vi "Save_to_Project.vi"(8 "error in (no error)":errorcluster, 9 "index":string, 10 "buildObject":T1, 11 "absFolder in":refnum<class "absFolder.lvclass">) -> (0 "error out":errorcluster, 1 "index out":string, 2 "buildObject out":T1, 3 "absFolder out":refnum<class "absFolder.lvclass">, 5 "saved?":bool)   [LabVIEW 2020, in "absFolder.lvclass"]
uses:
  <vilib>/AppBuilder/IB_Classes/Destination/absFolder/absFolder.lvclass
  <vilib>/AppBuilder/IB_Classes/Destination/absFolder/absFolder.lvclass/absFolder.ctl
  <vilib>/AppBuilder/IB_Classes/Destination/IB_Destination.lvclass
  <vilib>/AppBuilder/IB_RW_Project/IB_RW_Project_PropBag_Action.ctl
  <resource>/Framework/Providers/API/ItemRef.ctl
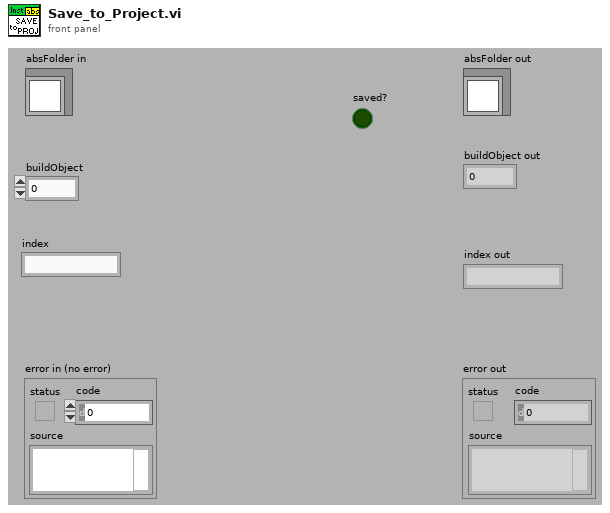
[diagram p1: front panel]
types:
  T1 = typedef "ItemRef.ctl" = u64
  T2 = typedef "IB_RW_Project_PropBag_Action.ctl" = enum16{"read", "write", "clear", "readPrevious", "writePrevious", "clearPrevious"}
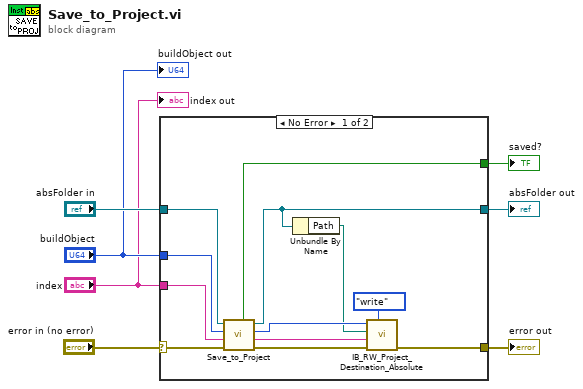
[diagram p0: block diagram]
diagram:
  n1 = case shown="No Error" "error in (no error)" {
    selector: "error in (no error)" -> [w8 w21]
    tunnel: [w19 _] -> w7
    tunnel: "index" -> [w18 _]
    tunnel: "buildObject" -> [w17 _]
    tunnel: "absFolder in" -> [w16 w20]
    tunnel: [w15 w20] -> w5
    tunnel: [w12 w21] -> w4
    frame No Error {
      n2 = call-parent "Save_to_Project.vi"("error in (no error)"=w8, "index"=w18, "buildObject"=w17, "IB_Destination in"=w16) -> ("error out"=w13:errorcluster, "index out"=w10:string, "buildObject out"=w11:T1, "IB_Destination out"=w15:refnum<class "absFolder.lvclass">, "saved?"=w19:bool)  [unwired: 3 in]
      n3 = Unbundle By Name(w15) -> ("Path"=w9:path)
      n4 = call <vilib>:"IB_RW_Project_Destination_Absolute.vi"("action"=IB_RW_Project_PropBag_Action."write", "ErrIn"=w13, "index"=w10, "Path"=w9, "buildObject"=w11) -> ("ErrOut"=w12:errorcluster)  [unwired: 3 in, 3 out]
    }
    frame Error {
    }
  }
  "error out" <- w4
  "absFolder out" <- w5
  "saved?" <- w7
  "buildObject out" <- "buildObject"
  "index out" <- "index"
